vi "Values String Mouse Down.vi"(8 "error in (no error)":errorcluster, 10 "Coords":T1, 11 "Application Data in":T2={"Item Tree Control"=refnum, "Top-Level VI"=refnum, "menu reference"=refnum, "queue"=refnum, "Stop Pointer"=refnum, "Buffer Variant"=variant, "server ID"=refnum, "framework tag"="", "Values"=refnum, "Hex"=refnum, "ASCII"=refnum, "lines visible"=0, "values padding"=0, "current buffer data"={"decimation"=0, "avg bandwidth"=0.0, "channels"=[], "byte order"=enum."little-endian", "buffer descriptor"={"buffer type"=enum."Engine", "plugin id"=0, "group id"=0, "transfer id"=0, "offset"=0, "length"=0}, "values channels"={"index"=0, "count"=0, "engine offset"=0}, "select start offset"=18446744073709551615, "select end offset"=0, "channel index"=-1}, "Framework Configuration"=refnum} {"current buffer data"."channels"."configuration"."string offset" format="%d bytes"; "current buffer data"."avg bandwidth" format="%.0g bytes"}) -> (0 "error out":errorcluster, 3 "Application Data out":T2={"Item Tree Control"=refnum, "Top-Level VI"=refnum, "menu reference"=refnum, "queue"=refnum, "Stop Pointer"=refnum, "Buffer Variant"=variant, "server ID"=refnum, "framework tag"="", "Values"=refnum, "Hex"=refnum, "ASCII"=refnum, "lines visible"=0, "values padding"=0, "current buffer data"={"decimation"=0, "avg bandwidth"=0.0, "channels"=[], "byte order"=enum."little-endian", "buffer descriptor"={"buffer type"=enum."Engine", "plugin id"=0, "group id"=0, "transfer id"=0, "offset"=0, "length"=0}, "values channels"={"index"=0, "count"=0, "engine offset"=0}, "select start offset"=18446744073709551615, "select end offset"=0, "channel index"=-1}, "Framework Configuration"=refnum} {"current buffer data"."channels"."configuration"."string offset" format="%d bytes"; "current buffer data"."avg bandwidth" format="%.0g bytes"})   [LabVIEW 2021, in "DSF Core.lvlib"]
uses:
  DSF Core.lvlib
  Application Data.ctl
  <vilib>/NI/Memory Manager/Classes/Pointer/Pointer.lvclass
  Classes/Configuration/Core/Framework/Framework Configuration.lvclass
  Buffer Reader/Queue Data.ctl
  Buffer Reader/Buffer Data.ctl
  Classes/Configuration/Core/Transfer/Channel Configuration.ctl
  Typedefs/Core Channel Configuration.ctl
  Typedefs/DSF Data Type.ctl
  Typedefs/DSF Settings Info.ctl
  Typedefs/DSF Byte Order.ctl
  Classes/Thread/Data Server/DSF Buffer Subset Descriptor.ctl
  Typedefs/DSF Buffer Type.ctl
  Values Channels.ctl
  <vilib>/Utility/miscctls.llb/LVPoint32TypeDef.ctl
  Classes/Framework/Framework.lvclass
  Classes/Configuration/Core/Channel/Channel Configuration.lvclass
  Classes/Configuration/Core/Transfer/Transfer Configuration.lvclass
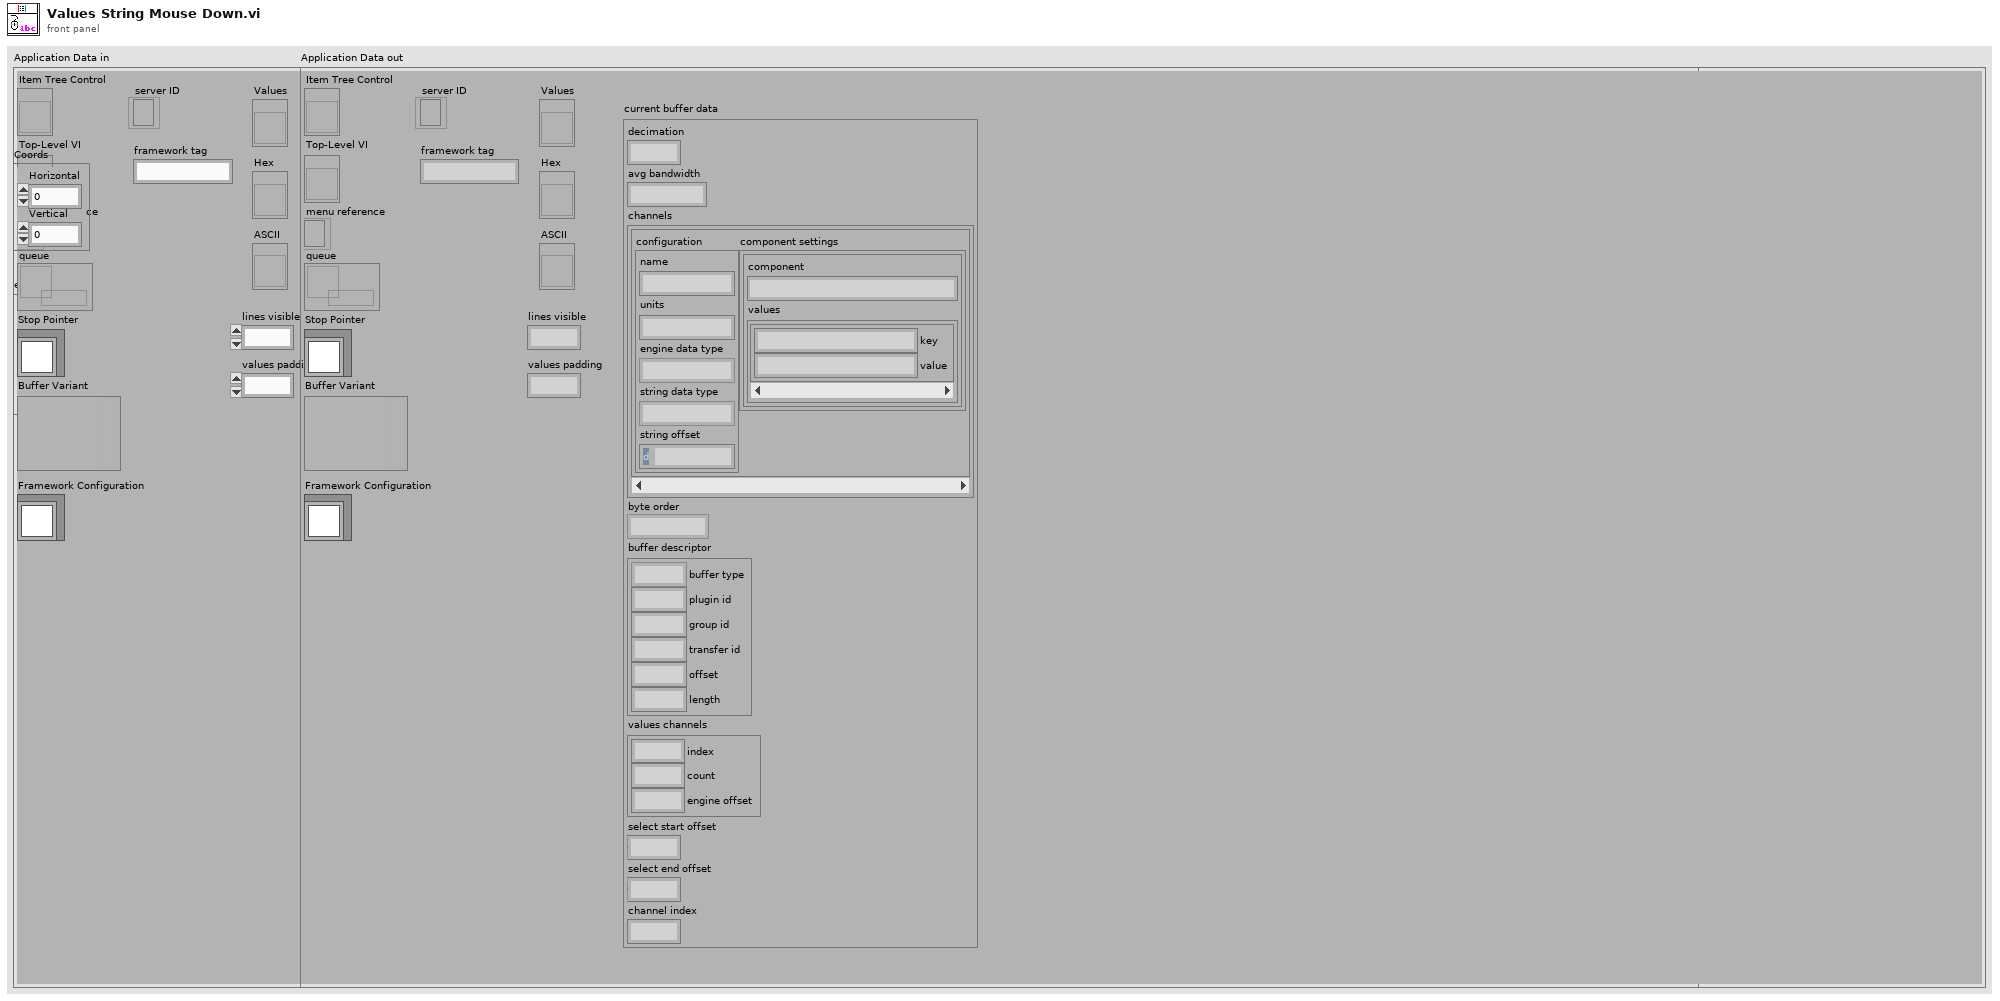
[diagram p1: front panel]
types:
  T1 = typedef "LVPoint32TypeDef.ctl" = cluster{"Horizontal":i32, "Vertical":i32}
  T2 = typedef "DSF Core.lvlib/Application Data.ctl" = cluster{"Item Tree Control":refnum<vi>, "Top-Level VI":refnum<vi>, "menu reference":refnum<k9>, "queue":refnum<queue>, "Stop Pointer":refnum<class "Pointer.lvclass">, "Buffer Variant":variant, "server ID":refnum<k5>, "framework tag":string, "Values":refnum<vi>, "Hex":refnum<vi>, "ASCII":refnum<vi>, "lines visible":i32, "values padding":i32, "current buffer data":T3, "Framework Configuration":refnum<class "Framework Configuration.lvclass">}
  T3 = typedef "DSF Core.lvlib/Buffer Data.ctl" = cluster{"decimation":u64, "avg bandwidth":dbl, "channels":T4[], "byte order":T8, "buffer descriptor":T9, "values channels":T11, "select start offset":u64, "select end offset":u64, "channel index":i32}
  T4 = typedef "DSF Core.lvlib/Transfer Configuration.lvclass/Channel Configuration.ctl" = cluster{"configuration":T5, "component settings":T7[]}
  T5 = typedef "DSF Core.lvlib/Channel Configuration.lvclass/Core Channel Configuration.ctl" = cluster{"name":string, "units":string, "engine data type":T6, "string data type":T6, "string offset":u64}
  T6 = typedef "DSF Core.lvlib/DSF Data Type.ctl" = enum8{"Bool", "SGL", "DBL", "I8", "I16", "I32", "I64", "U8", "U16", "U32", "U64"}
  T7 = typedef "DSF Core.lvlib/DSF Settings Info.ctl" = cluster{"component":string, "values":cluster{"key":string, "value":string}[]}
  T8 = typedef "DSF Core.lvlib/DSF Byte Order.ctl" = enum8{"big-endian", "little-endian"}
  T9 = typedef "DSF Core.lvlib/DSF Buffer Subset Descriptor.ctl" = cluster{"buffer type":T10, "plugin id":i32, "group id":i32, "transfer id":i32, "offset":u64, "length":i64}
  T10 = typedef "DSF Core.lvlib/DSF Buffer Type.ctl" = enum16{"Engine", "String"}
  T11 = typedef "DSF Core.lvlib/Values Channels.ctl" = cluster{"index":i32, "count":i32, "engine offset":u64}
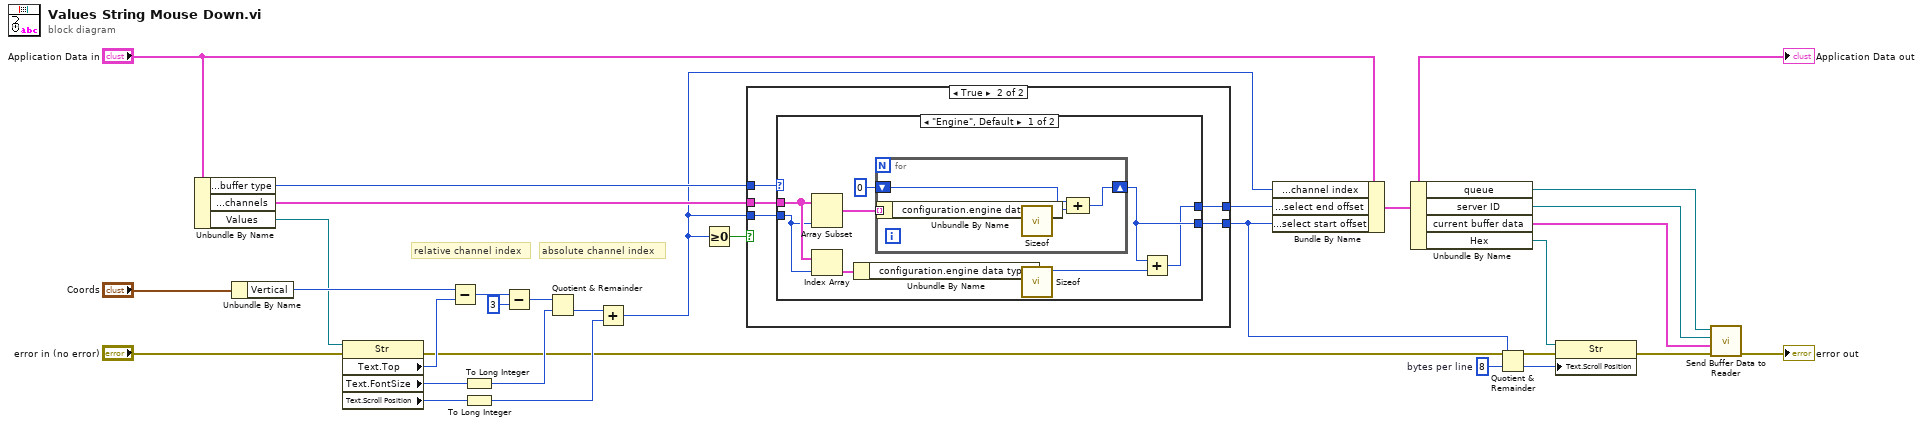
[diagram p0: block diagram]
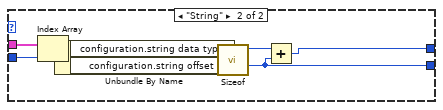
[diagram p3: hidden frame]
diagram:
  w3 = u64 8  # bytes per line
  # "absolute channel index"
  # "relative channel index"
  n1 = Unbundle By Name("Application Data in") -> ("current buffer data.buffer descriptor.buffer type"=w20:T10, "current buffer data.channels"=w18:T4[], "Values"=w21:refnum<vi>)
  n2 = Unbundle By Name("Coords") -> ("Vertical"=w23:i32)
  n3 = property class="Str"(reference=w21, error in="error in (no error)") -> (error out=w5:errorcluster, "Text.Top"=w17:i32, "Text.FontSize"=w25:u32, "Text.Scroll Position"=w24:u32)  [unwired: 1 out]
  n4 = Subtract(x=w23, y=w17) -> (x-y=w28:i32)
  n5 = To Long Integer(number=w25) -> (32bit integer=w16:i32)
  n6 = To Long Integer(number=w24) -> (32bit integer=w15:i32)
  n7 = Subtract(x=w28, y=3) -> (x-y=w26:i32)
  n8 = Quotient & Remainder(x=w26, y=w16) -> (floor(x/y)=w22:i32)  [unwired: 1 out]
  n9 = Add(x=w22, y=w15) -> (x+y=w7:i32)
  n10 = Greater Or Equal To 0?(x=w7) -> (x >= 0?=w19:bool)
  n11 = case shown="True" w19 {
    tunnel: w18 -> [_ w32]
    tunnel: w20 -> [_ w35]
    tunnel: w7 -> [_ w31]
    tunnel: [_ w34] -> w2
    tunnel: [_ w33] -> w14
    frame False {
    }
    frame True {
      n12 = case shown="\"Engine\", Default" w35 {
        tunnel: [w38 w51] -> w34
        tunnel: [w37 w50] -> w33
        tunnel: w32 -> [w42 w55]
        tunnel: w31 -> [w41 w54]
        frame "Engine", Default {
          n13 = Array Subset(array=w42, length=w41) -> (w44:T4[])  [unwired: 1 in]
          n14 = Index Array(array=w42, index=w41) -> (element=w40:T4)
          n15 = Unbundle By Name(w40) -> ("configuration.engine data type"=w39:T6)
          n16 = for {
            tunnel: w44 -> [w49] mode=indexing
            shift-right: [w46] -> w38
            shift-left: u64 0 -> [w45]
            n17 = Unbundle By Name(w49) -> ("configuration.engine data type"=w48:T6)
            n18 = call "Sizeof.vi"("data type"=w48) -> ("size in bytes"=w47:u64)  [unwired: 9 in, 1 out]
            n19 = Compound Arithmetic op=ADD(w45, w47) -> (w46:u64)
          }
          n20 = call "Sizeof.vi"("data type"=w39) -> ("size in bytes"=w36:u64)  [unwired: 9 in, 1 out]
          n21 = Add(x=w38, y=w36) -> (x+y=w37:u64)
        }
        frame "String" {
          n22 = Index Array(array=w55, index=w54) -> (element=w53:T4)
          n23 = Unbundle By Name(w53) -> ("configuration.string data type"=w56:T6, "configuration.string offset"=w51:u64)
          n24 = call "Sizeof.vi"("data type"=w56) -> ("size in bytes"=w52:u64)  [unwired: 9 in, 1 out]
          n25 = Add(x=w52, y=w51) -> (x+y=w50:u64)
        }
      }
    }
  }
  n26 = Bundle By Name(cluster="Application Data in", "current buffer data.channel index"=w7, "current buffer data.select end offset"=w14, "current buffer data.select start offset"=w2) -> (w8:T2)
  "Application Data out" <- w8
  n27 = Unbundle By Name(w8) -> ("queue"=w9:refnum<queue>, "server ID"=w10:refnum<k5>, "current buffer data"=w11:T3, "Hex"=w6:refnum<vi>)
  n28 = Quotient & Remainder(x=w2, y=w3) -> (floor(x/y)=w1:u64)  [unwired: 1 out]
  n29 = property class="Str"(reference=w6, error in=w5, "Text.Scroll Position"=w1) -> (error out=w4:errorcluster)  [unwired: 1 out]
  n30 = call "Send Buffer Data to Reader.vi"("error in (no error)"=w4, "Buffer data"=w11, "server ID"=w10, "queue"=w9) -> ("error out"=→"error out":errorcluster)  [unwired: 7 in]
